vi "controlLaw_delay_Integral_trackTraj.vi"(7 "Cluster":T1={"umax"=3.0, "y_ref(k)"=0.0, "Ki"=0.0, "y(k) (from plant)"=0.0, "ND"=0, "NS"=0, "u_Kx_ref(k)"=0.0} {"u_Kx_ref(k)" format="%#_13g"; "Ki" format="%#_13g"; "y_ref(k)" format="%#_13g"; "umax" format="%#_13g"}, 8 "Xd_in":T2=[0.0, 0.0, 0.0, 0.0, 0.0, 0.0, 0.0, 0.0, 0.0, 0.0, 0.0, 0.0], 9 "x^(k)":sgl[](array[numeric])=[0.0, 0.0, 0.0, 0.0, 0.0, 0.0, 0.0, 0.0, 0.0, 0.0, 0.0, 0.0, 0.0, 0.0, 0.0, 0.0, 0.0, 0.0, 0.0, 0.0, 0.0, 0.0, 0.0, 0.0, 0.0]) -> (0 "Xd_out(k+1)":T2 caption="Xd_out", 1 "x^(k+1) = Ax + Bu + Lye":sgl[](array[numeric]), 4 "u(k) (saturated)":sgl)   [LabVIEW 2017]
uses:
  controls/Xdelay.ctl
  <vilib>/Platform/TimedLoop/XDataNode/timing_clust.ctl
  <vilib>/Platform/TimedLoop/XDataNode/nitl_modes.ctl
  <vilib>/Platform/TimedLoop/XDataNode/wakeup.ctl
  <vilib>/rvi/DataTransferAndStorage/Container/Common/niFpgaContainerExecOnDevCompGetState.vi
  <vilib>/rvi/Emulation/niFpgaEmulationIsFPGAContextNoSignature.vi
  <vilib>/rvi/DataTransferAndStorage/Container/Common/niFpgaContainerGetUniqueNameForEmu.vi
  <vilib>/rvi/Memory/Memory_Emulation/niFpgaMemoryEmulationCacheClearOnFirstRun.vi
  <vilib>/rvi/Memory/Memory_Emulation/nirvimemoryEmulationManagerCache_MakeExclusive.vi
  <vilib>/rvi/Memory/Memory_Emulation/niFpgaMemoryEmulationValidateCache.vi
  <vilib>/rvi/Memory/Memory_Emulation/nirvimemoryEmulationManagerCache_InsertValue.vi
  <vilib>/Utility/error.llb/Clear Errors.vi
  <vilib>/rvi/Memory/Memory_Emulation/nirvimemoryEmulationManagerCache_ReleaseExclusive.vi
  <vilib>/rvi/Memory/Memory_Emulation/nirvimemoryEmulationManagerCache_GetValue.vi
  <vilib>/rvi/Memory/Memory_Emulation/nirvimemoryEmulationManagerCache_SetValue.vi
  <vilib>/rvi/Emulation/niFpgaProcessEmulError.vi
  <vilib>/rvi/Emulation/niFpgaSctlEmulationGetInTimedLoop.vi
  <vilib>/rvi/Emulation/niFpgaEmulationReportErrorSimple.vi
  <vilib>/rvi/Emulation/niFpgaGetClockAttributes.vi
  <vilib>/rvi/Emulation/niFpgaCriticalErrorInLSC.vi
  <vilib>/Platform/TimedLoop/XDataNode/XDataNode.xnode
  <vilib>/rvi/DataTransferAndStorage/Container/XNode/niFpgaContainer.xnode
  <vilib>/rvi/DataTransferAndStorage/Register/Emulation/niFpgaRegisterEmulationRefIn.vi
  <vilib>/Platform/TimedLoop/XDataNode/XDNodeRunTimeDep.lvlib
panel:
  out "u = -Kx + Nbar*r":sgl format="%#_13g"
  out "-K*x(k)":sgl format="%#_13g"
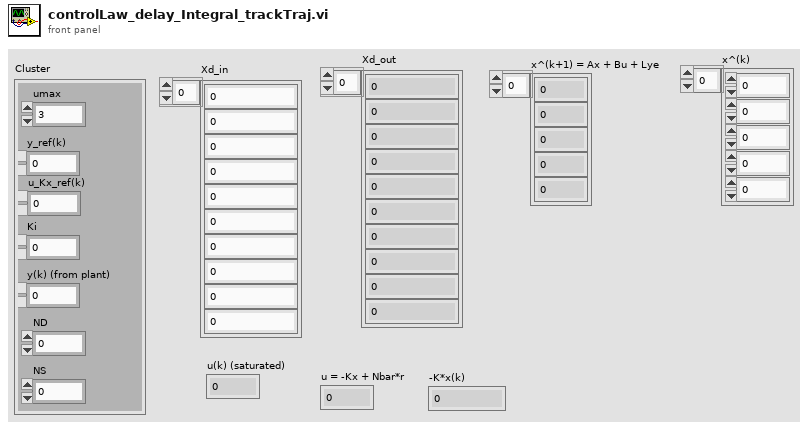
[diagram p1: front panel]
types:
  T1 = cluster{"umax":sgl, "y_ref(k)":sgl, "Ki":sgl, "y(k) (from plant)":sgl, "ND":i16, "NS":i16, "u_Kx_ref(k)":sgl}
  T2 = typedef "Xdelay.ctl" = sgl[]
  T3 = typedef "XDNodeRunTimeDep.lvlib/timing_clust.ctl" = cluster{"Expected End [f-1]":u64, "Actual End [f-1]":u64, "Finished Late? [f-1]":bool, "Expected End [i-1]":u64, "Actual End [i-1]":u64, "Finished Late? [i-1]":bool, "Expected Start [i]":u64, "Actual Start [i]":u64, "Expected Start [f]":u64, "Actual Start [f]":u64, "Source Name":string, "Structure Name":string, "Period":i64, "Deadline":i64, "Offset":i64, "Start":i64, "Priority":i32, "Timeout":i32, "Mode":T4, "Wakeup Reason":T5, "Error":errorcluster, "Source Type":string, "Secondary Source Type":string, "Global End Time":u64, "Global Start Time":u64, "Frame Duration":u64, "Iteration Duration":u64, "Assigned CPU":i32, "I/O Scan Engine Mode":u32}
  T4 = typedef "XDNodeRunTimeDep.lvlib/nitl_modes.ctl" = enum32{"No Change", "Process missed periods, maintain original phase", "Discard missed periods, maintain original phase", "Process missed periods, ignore original phase", "Discard missed periods, ignore original phase"}
  T5 = typedef "XDNodeRunTimeDep.lvlib/wakeup.ctl" = enum32{"Normal", "Aborted", "Asynchronous wakeup", "Timing source error", "Timed loop error", "Timeout"}
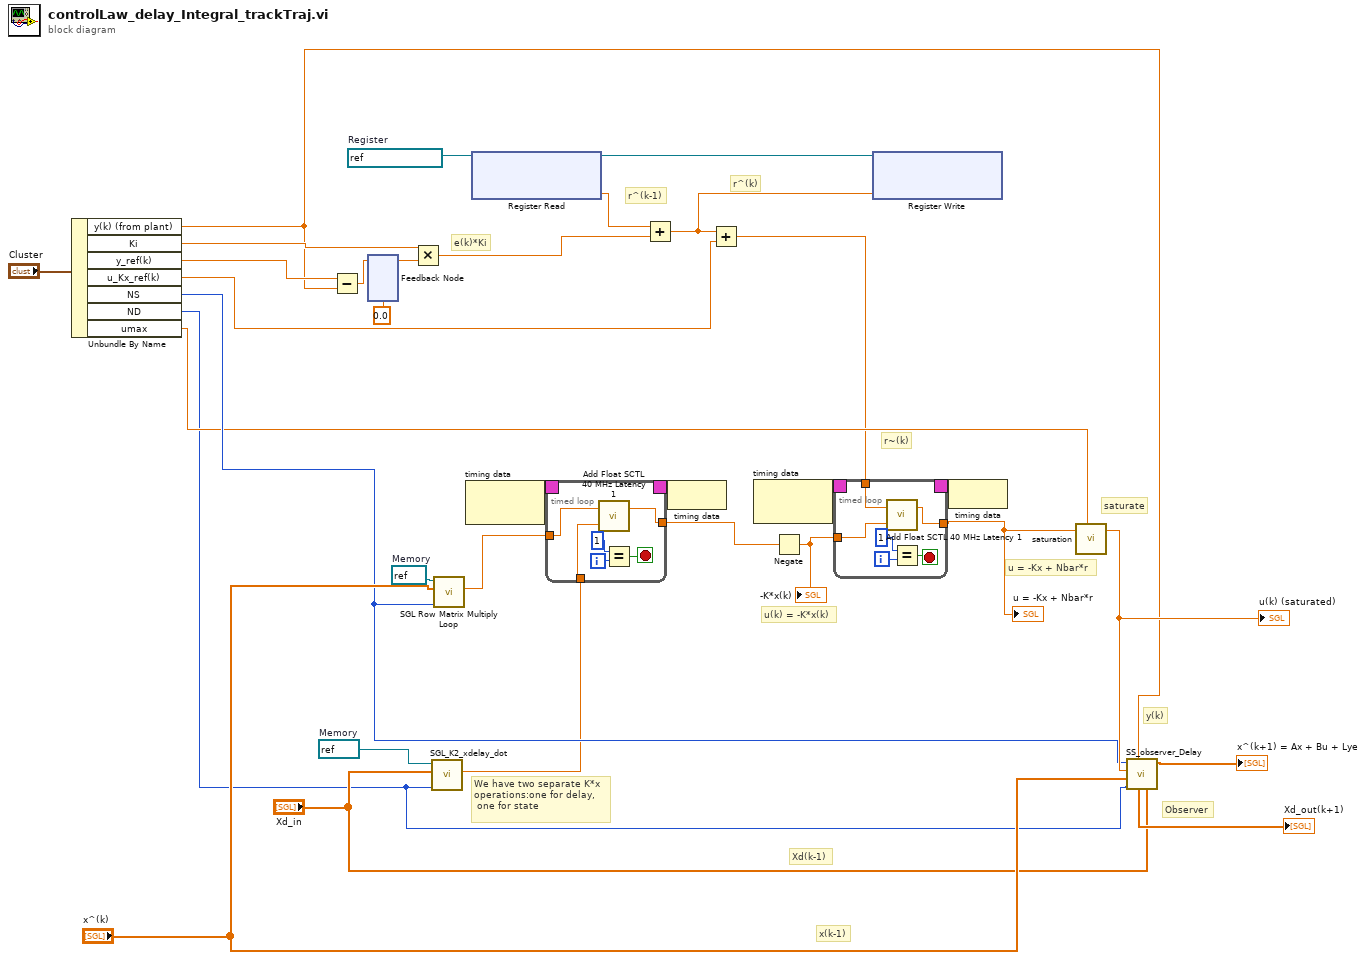
[diagram p0: block diagram]
diagram:
  w20 = refnum<k21> "accumulator"  # Register
  w8 = refnum<k21> "K2"  # Memory
  w25 = refnum<k21> "K"  # Memory
  # "y(k)"
  # "Xd(k-1)"
  # "x(k-1)"
  # "r^(k)"
  # "r^(k-1)"
  # "e(k)*Ki"
  # "r~(k)"
  # "We have two separate K*x\noperations:one for delay,\n one for state"
  # "saturate"
  # "u = -Kx + Nbar*r"
  # "u(k) = -K*x(k)"
  # "Observer"
  n1 = Unbundle By Name("Cluster") -> ("y(k) (from plant)"=w11:sgl, "Ki"=w14:sgl, "y_ref(k)"=w12:sgl, "u_Kx_ref(k)"=w2:sgl, "NS"=w13:i16, "ND"=w6:i16, "umax"=w10:sgl)
  n2 = Subtract(x=w12, y=w11) -> (x-y=w4:sgl)
  n3 = feedback #1(sgl 0.0) -> (w5:sgl)
  n4 = feedback-in #1(w4) -> ()
  n5 = Multiply(x=w14, y=w5) -> (x*y=w22:sgl)
  n6 = call "SGL_K2_xdelay_dot.vi"("ND"=w6, "X"="Xd_in", "Refnum in"=w8) -> ("Numeric"=w9:sgl)  [unwired: 8 in]
  n7 = call "SGL Row Matrix Multiply Loop.vi"("NS"=w13, "X"="x^(k)", "Refnum in"=w25) -> ("Numeric"=w28:sgl)  [unwired: 8 in]
  n8 = node-c288() -> (w31:T3)  [unwired: 1 in]
  n9 = xnode ("Register Read")("Register In"=w20) -> ("Data"=w23:sgl, "Register Out"=w24:refnum<k21>)
  n10 = timed-loop {
    timing: w31 -> [_]
    timing-out: [_] -> w30
    tunnel: w28 -> [w34]
    tunnel: [w39] -> w27
    tunnel: w9 -> [w38]
    i -> [w35]
    stop <- w37 stop-if-true
    n11 = call "Add Float SCTL 40 MHz Latency 1.vi"("y"=w38, "x"=w34) -> ("x[k-1]+y[k-1]"=w39:sgl)  [unwired: 1 out]
    n12 = Equal?(x=i16 1, y=w35) -> (x = y?=w37:bool)
  }
  n13 = Add(x=w23, y=w22) -> (x+y=w21:sgl)
  n14 = node-c288(w30) -> ()
  n15 = Add(x=w21, y=w2) -> (x+y=w1:sgl)
  n16 = node-c288() -> (w33:T3)  [unwired: 1 in]
  n17 = Negate(x=w27) -> (-x=w26:sgl)
  "-K*x(k)" <- w26
  n18 = timed-loop {
    timing: w33 -> [_]
    timing-out: [_] -> w32
    tunnel: w1 -> [w47]
    tunnel: w26 -> [w46]
    tunnel: [w42] -> w29
    i -> [w43]
    stop <- w45 stop-if-true
    n19 = call "Add Float SCTL 40 MHz Latency 1.vi"("y"=w46, "x"=w47) -> ("x[k-1]+y[k-1]"=w42:sgl)  [unwired: 1 out]
    n20 = Equal?(x=i16 1, y=w43) -> (x = y?=w45:bool)
  }
  "u = -Kx + Nbar*r" <- w29
  n21 = xnode ("Register Write")("Data"=w21, "Register In"=w24) -> ()  [unwired: 1 out]
  n22 = node-c288(w32) -> ()
  n23 = call "saturation.vi"("uMax"=w10, "signal in"=w29) -> ("signal out"=w18:sgl)  [unwired: 9 in]
  "u(k) (saturated)" <- w18
  n24 = call "SS_observer_Delay.vi"("Xd_in"="Xd_in", "y(k)"=w11, "Nd"=w6, "X"="x^(k)", "u(predelay)(k)"=w18, "NS"=w13) -> ("Ax + Bu + Lye"=→"x^(k+1) = Ax + Bu + Lye":sgl[], "Xd_out"=→"Xd_out(k+1)":T2)  [unwired: 4 in]
